vi "DSF.Execution.Runtime.Plugin Manager.Query Disk.Classes.vi"(8 "error in (no error)":errorcluster, 10 "folder":path, 11 "Plugin Manager in":refnum<class "DSF.Engine.Runtime.Plugin Manager.lvclass">) -> (0 "error out":errorcluster, 2 "class paths":path[](array[path]), 3 "Plugin Manager out":refnum<class "DSF.Engine.Runtime.Plugin Manager.lvclass">)   [LabVIEW 2016, in "DSF.Engine.lvlib" / "DSF.Engine.Runtime.Plugin Manager.lvclass"]
uses:
  DSF.Engine.Runtime.Plugin Manager.lvclass
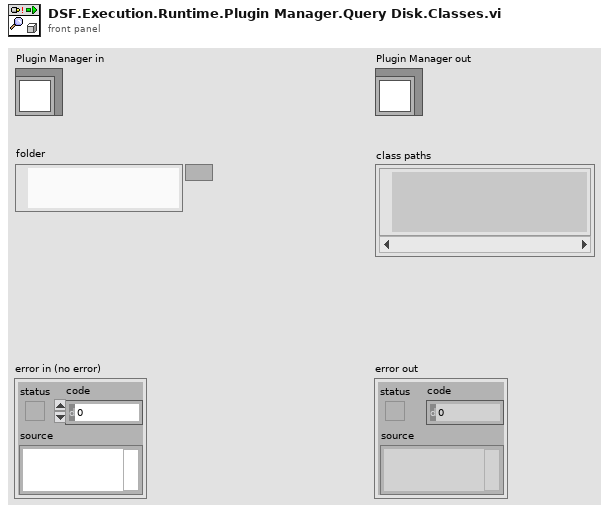
[diagram p1: front panel]
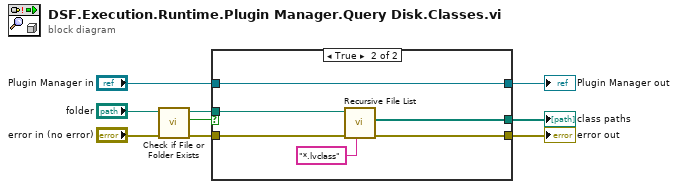
[diagram p0: block diagram]
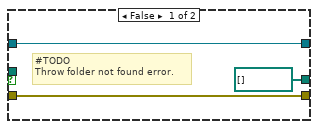
[diagram p2: hidden frame]
diagram:
  n1 = call <vilib>:"Check if File or Folder Exists.vi"("error in (no error)"="error in (no error)", "path"="folder") -> ("error out"=w8:errorcluster, "file or folder exists?"=w9:bool, "dup path"=w7:path)  [unwired: 7 in]
  n2 = case shown="True" w9 {
    tunnel: w8 -> [w12 w16]
    tunnel: w7 -> [_ w17]
    tunnel: [w12 w15] -> w4
    tunnel: [path[] [] ("All Files in Dir") w14] -> w6
    tunnel: "Plugin Manager in" -> [w10 w13]
    tunnel: [w10 w13] -> w1
    frame False {
      # "#TODO\nThrow folder not found error."
    }
    frame True {
      n3 = call <vilib>:"Recursive File List.vi"("pattern"="*.lvclass", "error in (no error)"=w16, "Folder Path"=w17) -> ("error out"=w15:errorcluster, "All Files in Dir"=w14:path[])  [unwired: 4 in, 3 out]
    }
  }
  "error out" <- w4
  "Plugin Manager out" <- w1
  "class paths" <- w6
